vi "DSF.Engine.Runtime.Framework.Initialize Plugins.vi"(8 "error in (no error)":errorcluster, 11 "Framework Runtime in":refnum<class "DSF.Engine.Runtime.Framework.lvclass">) -> (0 "error out":errorcluster, 3 "Framework Runtime out":refnum<class "DSF.Engine.Runtime.Framework.lvclass">)   [LabVIEW 2016, in "DSF.Engine.lvlib" / "DSF.Engine.Runtime.Framework.lvclass"]
uses:
  DSF.Engine.Runtime.Framework.lvclass
  Plugin/DSF.Engine.Plugin.Runtime.lvclass
  DSF.Engine.Runtime.Framework.lvclass/DSF.Engine.Runtime.Framework.ctl
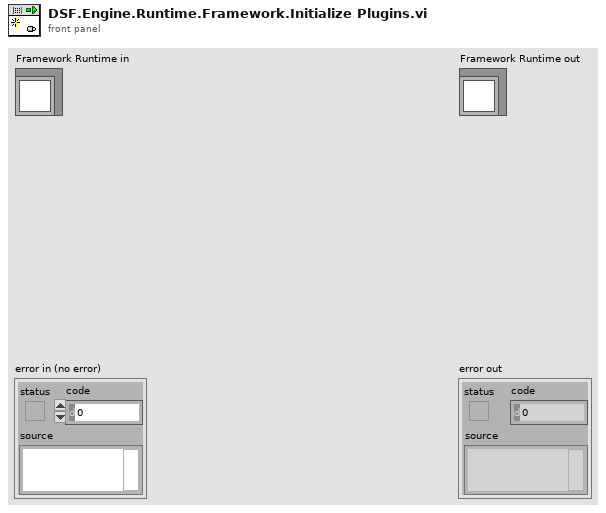
[diagram p1: front panel]
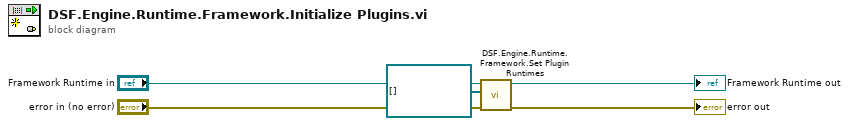
[diagram p0: block diagram]
diagram:
  n1 = call "DSF.Engine.Runtime.Framework.Set Plugin Runtimes.vi"("Plugin Runtimes"=refnum<class "DSF.Engine.Plugin.Runtime.lvclass">[] [], "Framework Runtime in"="Framework Runtime in") -> ("Framework Runtime out"=→"Framework Runtime out":refnum<class "DSF.Engine.Runtime.Framework.lvclass">)  [unwired: 9 in]
  "error out" <- "error in (no error)"
